vi "Navigation.vi"(0 "IA State Output in":T1, 7 "a1":dbl=10.0, 9 "a3":dbl=15.0, 11 "GoTo Navigation":bool, 12 "Debug":bool, 13 "output inc":dbl, 14 "output xy":dbl, 15 "output angle":dbl) -> (4 "IA State Output out":T1)   [LabVIEW 2018]
uses:
  Communication_class/Paths/MessageAI_State Folder/Intel/Command Enum.ctl
  Vision_class/Old vision/Controls/Functions Enum.ctl
  Utilities_class/Utilities.lvclass
  Vision_class/Old vision/Controls/AttackerStates.ctl
  Vision_class/Old vision/Controls/AI Robot.ctl
  Communication_class/Paths/MessageAI_State Folder/Core/AI Ball.ctl
  Communication_class/Paths/MessageAI_State Folder/Core/Field Size.ctl
  Communication_class/Paths/MessageAI_State Folder/Core/AI Judge.ctl
  Communication_class/Paths/MessageAI_State Folder/Util/Events/Events.ctl
  Communication_class/Paths/MessageAI_State Folder/Core/AI Input.ctl
  Vision_class/Old vision/Controls/PathDest.ctl
  Vision_class/Old vision/Controls/PathDests.ctl
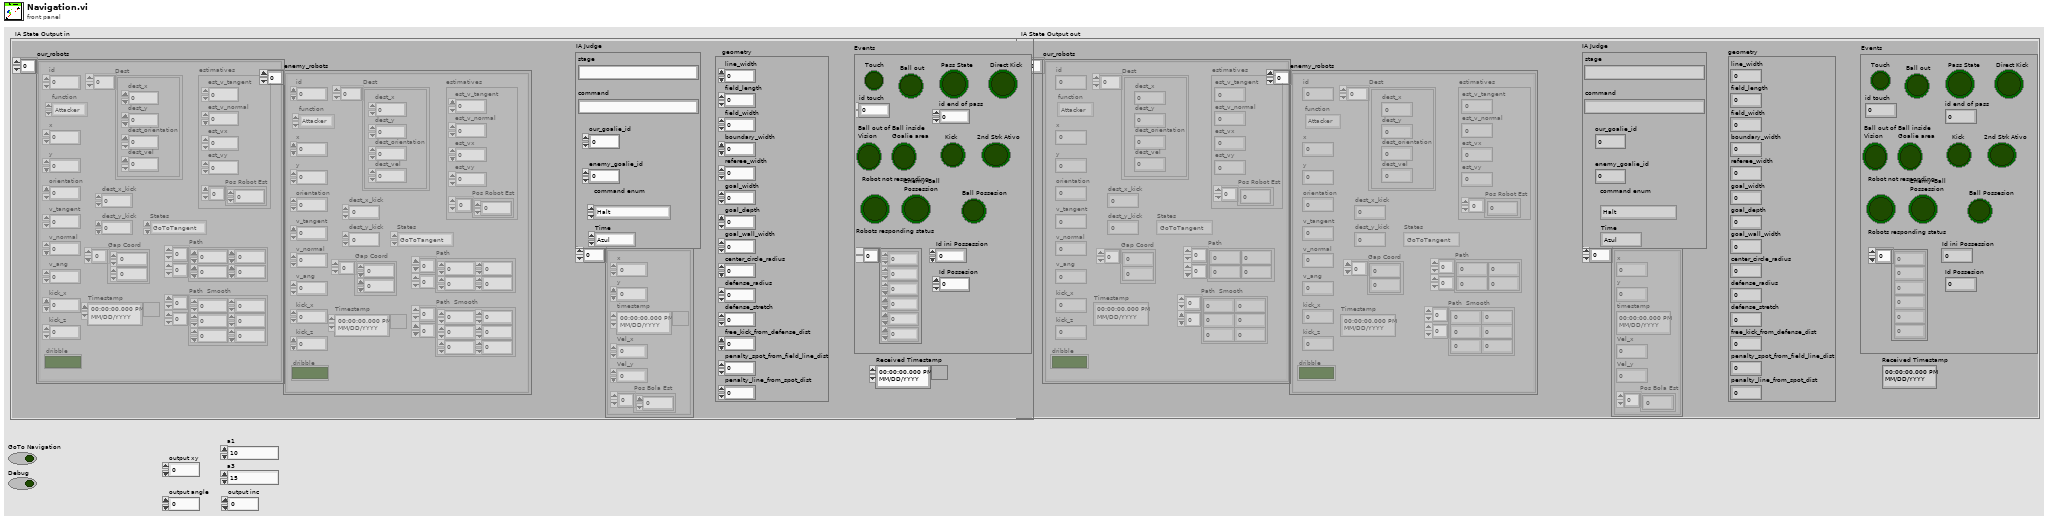
[diagram p1: front panel]
types:
  T1 = typedef "AI Input.ctl" = cluster{"our_robots":T2[], "enemy_robots":T2[], "balls":T7[], "geometry":T8, "IA Judge":T9, "Received Timestamp":timestamp, "Events":T11}
  T2 = typedef "AI Robot.ctl" = cluster{"id":u32, "function":T3, "x":dbl, "y":dbl, "orientation":dbl, "v_tangent":dbl, "v_normal":dbl, "v_ang":dbl, "kick_x":dbl, "kick_z":dbl, "dribble":bool, "Timestamp":timestamp, "estimatives":cluster{"est_v_tangent":dbl, "est_v_normal":dbl, "est_vx":dbl, "est_vy":dbl, "Pos Robot Est":dbl[]}, "dest_x_kick":dbl, "dest_y_kick":dbl, "Gap Coord":dbl[], "States":T4, "Path ":dbl[][], "Path  Smooth":dbl[][], "Dest":T5}
  T3 = typedef "Functions Enum.ctl" = enum16{"2nd Striker", "Attacker", "Goalie", "Defender", "Striker", "Goto 0", "Dummy", "Kicker", "ZigZag 0", "ZigZag 1", "ZigZag 2", "ZigZag 3", "ZigZag 4", "ZigZag 5", "ZigZag 6", "ZigZag 7", "ZigZag 8", ""}
  T4 = typedef "AttackerStates.ctl" = enum16{"Pass", "GoToTangent", "BallGetting", "GoToKick", ""}
  T5 = typedef "PathDests.ctl" = T6[]
  T6 = typedef "PathDest.ctl" = cluster{"dest_x":dbl, "dest_y":dbl, "dest_orientation":dbl, "dest_vel":dbl}
  T7 = typedef "AI Ball.ctl" = cluster{"x":dbl, "y":dbl, "timestamp":timestamp, "Vel_x":dbl, "Vel_y":dbl, "Pos Bola Est":dbl[]}
  T8 = typedef "Field Size.ctl" = cluster{"line_width":u32, "field_length":u32, "field_width":u32, "boundary_width":u32, "referee_width":u32, "goal_width":u32, "goal_depth":u32, "goal_wall_width":u32, "center_circle_radius":u32, "defense_radius":u32, "defense_stretch":u32, "free_kick_from_defense_dist":u32, "penalty_spot_from_field_line_dist":u32, "penalty_line_from_spot_dist":u32}
  T9 = typedef "AI Judge.ctl" = cluster{"stage":string, "command":string, "our_goalie_id":dbl, "enemy_goalie_id":dbl, "command enum":T10, "Time":enum16{"Azul", "Amarelo"}}
  T10 = typedef "Command Enum.ctl" = enum16{"Halt", "Stop", "Force Start", "PKA Normal Start", "Prepare Kickoff Ally", "PKE Normal Start", "Prepare Kickoff Enemy", "Prepare Penalty Ally", "PPA Normal Start", "Prepare Penalty Enemy", "PPE Normal Start", "Direct Free Enemy", "Direct Free Ally", "Indirect Free Enemy", "Indirect Free Ally", "Timeout Enemy", "Timeout Ally", "Goal Enemy", "Goal Ally", "Ball Placement Enemy", "Ball Placement Ally", "Normal Half Time", "Extra Time Break", "Extra Half Time", "None", "Post Game"}
  T11 = typedef "Events.ctl" = cluster{"Touch":bool, "Ball out":bool, "id touch":dbl, "Ball out of \nVision":bool, "Ball inside \nGoalie area":bool, "Robot not responding":bool, "Robots responding status":dbl[], "Enemy Ball \nPossession":bool, "Pass State":bool, "id end of pass":dbl, "Kick":bool, "Id ini Possession":dbl, "Ball Possesion":bool, "Id Possesion":dbl, "Direct Kick":bool, "2nd Strk Ativo":bool}
  T12 = cluster{"est_v_tangent":dbl, "est_v_normal":dbl, "est_vx":dbl, "est_vy":dbl, "Pos Robot Est":dbl[]}
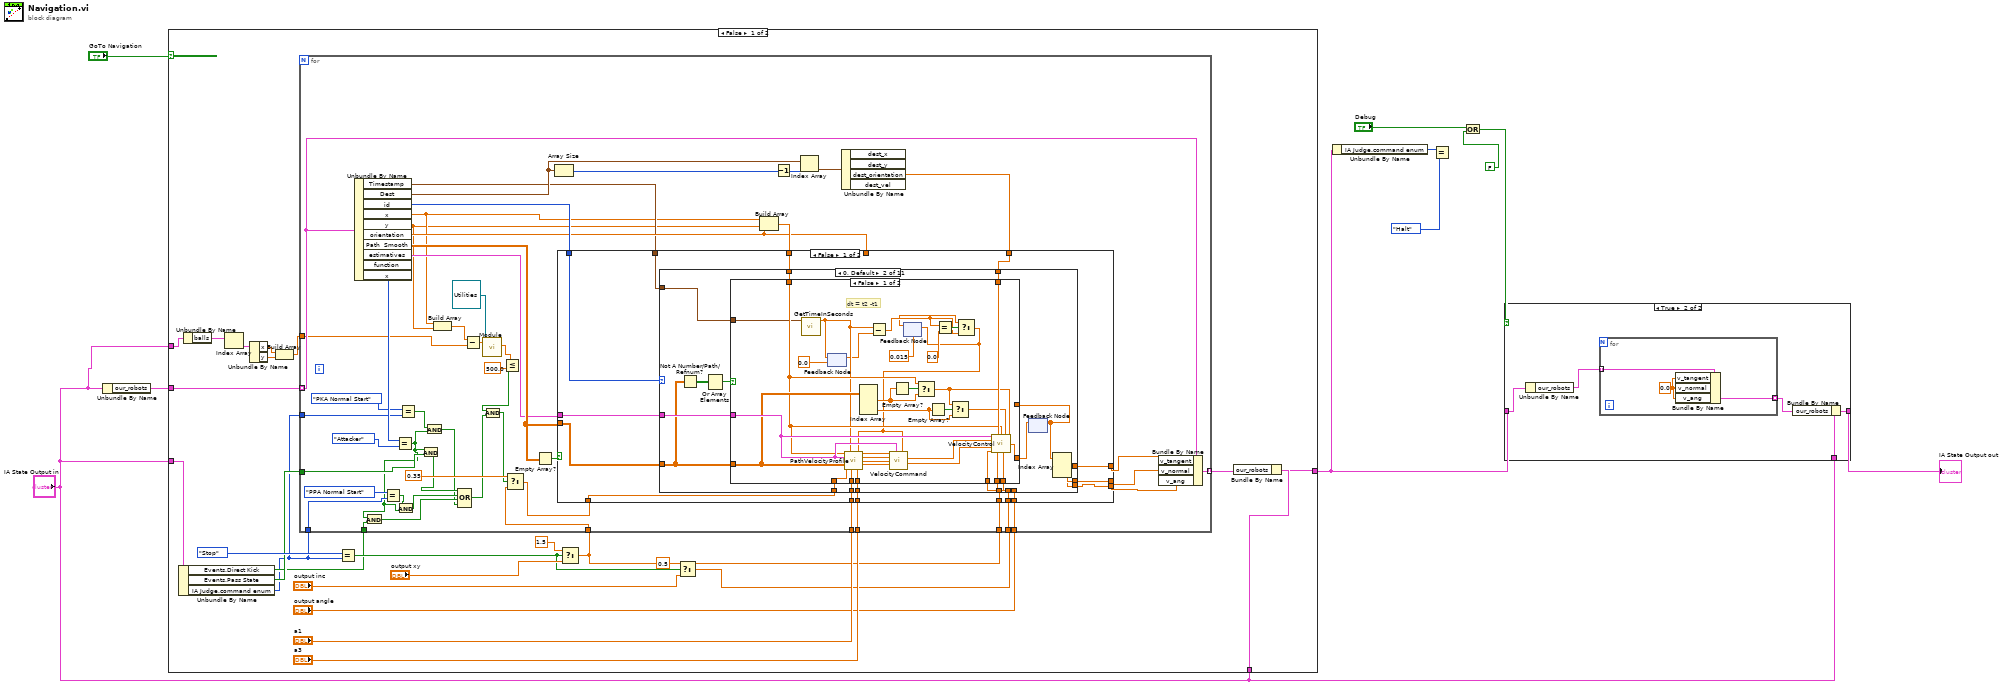
[diagram p0: block diagram]
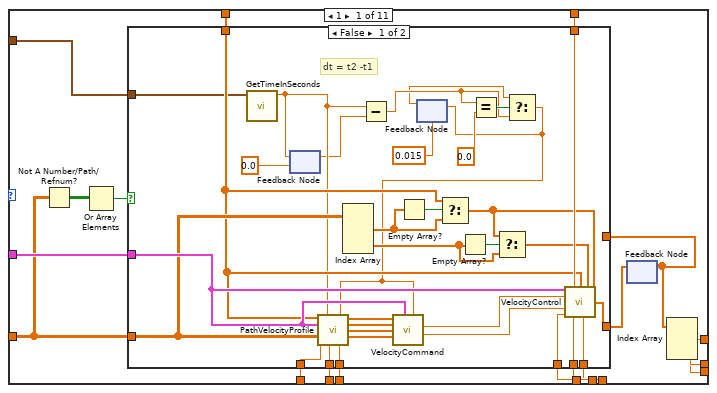
[diagram p2: hidden frame]
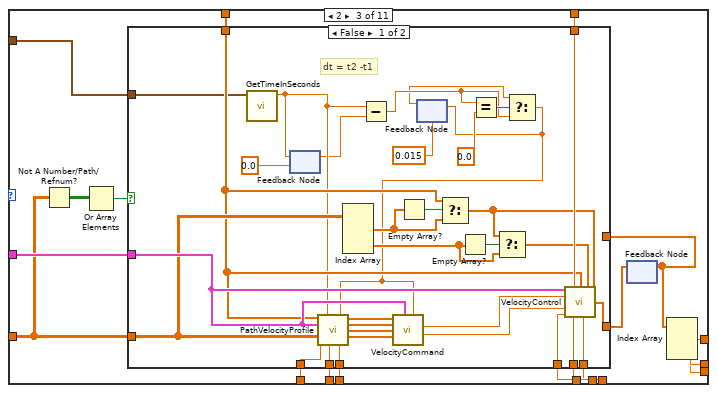
[diagram p5: hidden frame]
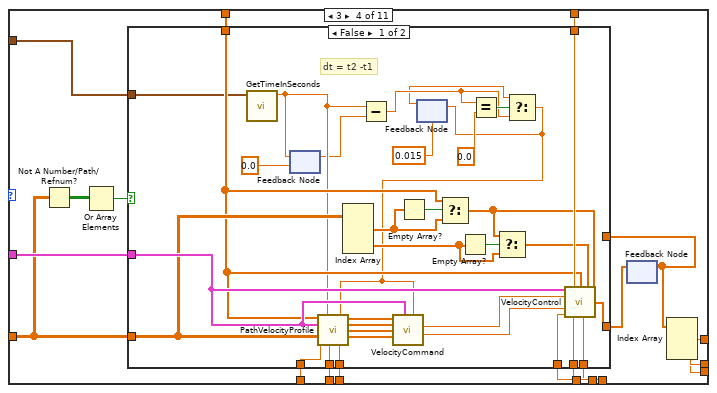
[diagram p7: hidden frame]
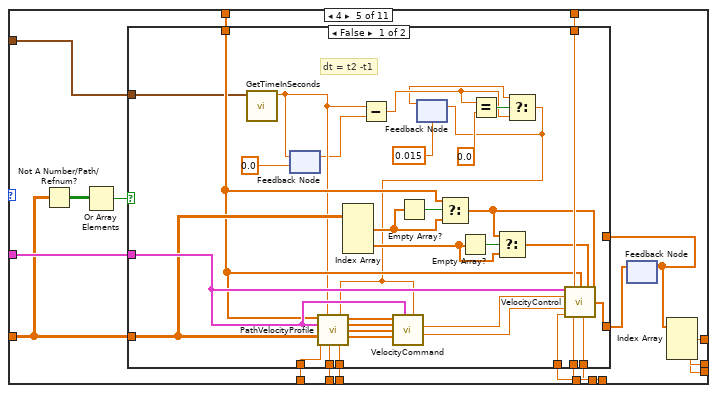
[diagram p9: hidden frame]
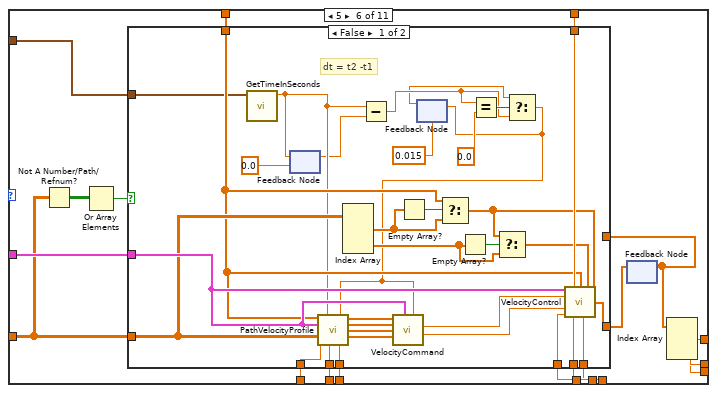
[diagram p11: hidden frame]
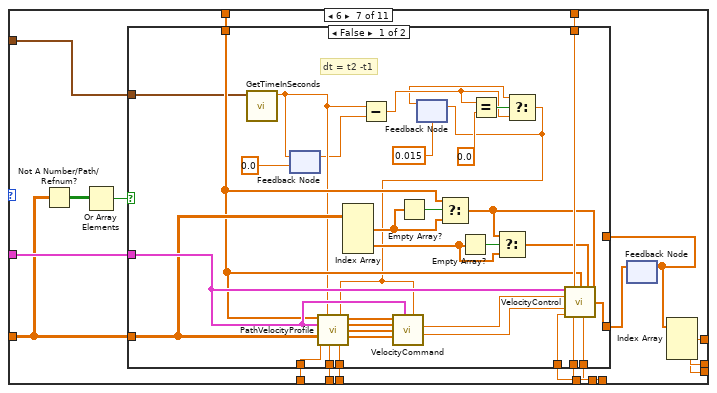
[diagram p13: hidden frame]
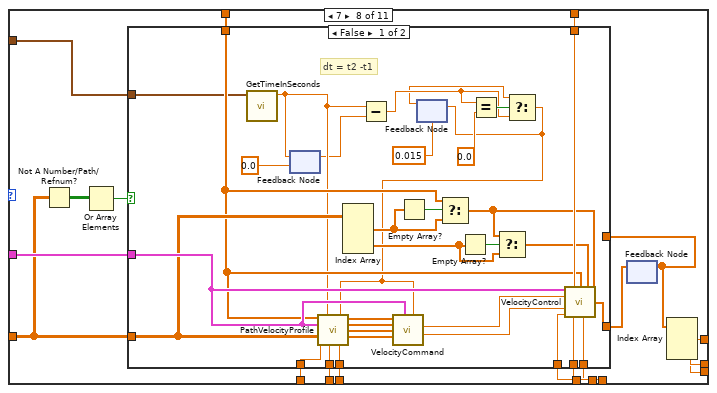
[diagram p15: hidden frame]
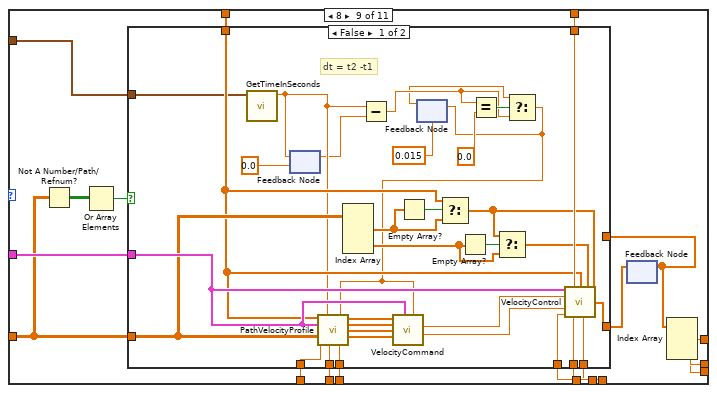
[diagram p17: hidden frame]
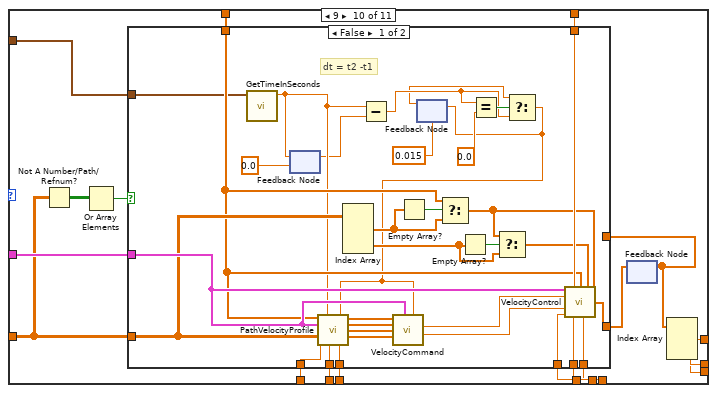
[diagram p19: hidden frame]
diagram:
  n1 = Unbundle By Name("IA State Output in") -> ("our_robots"=w10:T2[])
  n2 = case shown="False" "GoTo Navigation" {
    tunnel: w10 -> [w35 _]
    tunnel: [w32 w675] -> w7
    tunnel: "IA State Output in" -> [w28 w676]
    tunnel: "IA State Output in" -> [w33 _]
    tunnel: "IA State Output in" -> [w12 _]
    frame False {
      n3 = Unbundle By Name(w28) -> ("Events.Direct Kick"=w18:bool, "Events.Pass State"=w19:bool, "IA Judge.command enum"=w17:T10)
      n4 = Unbundle By Name(w12) -> ("balls"=w16:T7[])
      n5 = Index Array(array=w16) -> (element=w15:T7)  [unwired: 1 in]
      n6 = Unbundle By Name(w15) -> ("x"=w14:dbl, "y"=w13:dbl)
      n7 = Build Array(w14, w13) -> (w11:dbl[])
      n8 = Equal?(x=Command_Enum."Stop", y=w17) -> (x = y?=w23:bool)
      n9 = Select(t=1.5, s=w23, f="output xy") -> (s? t:f=w25:dbl)
      n10 = Select(t=0.5, s=w23, f="output inc") -> (s? t:f=w21:dbl)
      n11 = for {
        tunnel: w35 -> [w86] mode=indexing
        tunnel: [w85] -> w34 mode=indexing
        tunnel: w25 -> [w63]
        tunnel: "a1" -> [w74]
        tunnel: "a3" -> [w73]
        tunnel: w21 -> [w69]
        tunnel: "output angle" -> [w68]
        tunnel: w25 -> [w67]
        tunnel: w19 -> [w56]
        tunnel: w17 -> [w60]
        tunnel: w18 -> [w53]
        tunnel: w17 -> [w51]
        tunnel: w11 -> [w39]
        n12 = Unbundle By Name(w86) -> ("Timestamp"=w65:timestamp, "Dest"=w84:T5, "id"=w77:u32, "x"=w46:dbl, "y"=w45:dbl, "orientation"=w72:dbl, "Path  Smooth"=w78:dbl[][], "estimatives"=w75:T12, "function"=w52:T3)  [unwired: 1 out]
        n13 = Equal?(x=Command_Enum."PPA Normal Start", y=w60) -> (x = y?=w57:bool)
        n14 = Equal?(x=w52, y=Functions_Enum."Attacker") -> (x = y?=w48:bool)
        n15 = And(x=w48, y=w53) -> (x .and. y?=w54:bool)
        n16 = And(x=w57, y=w48) -> (x .and. y?=w55:bool)
        n17 = Equal?(x=Command_Enum."PKA Normal Start", y=w51) -> (x = y?=w49:bool)
        n18 = And(x=w48, y=w56) -> (x .and. y?=w58:bool)
        n19 = And(x=w49, y=w48) -> (x .and. y?=w47:bool)
        n20 = Build Array(w46, w45) -> (w40:dbl[])
        n21 = Compound Arithmetic op=OR(w58, w55, w54, w47) -> (w42:bool)
        n22 = Subtract(x=w40, y=w39) -> (x-y=w38:dbl[])
        n23 = call-dynamic "Module.vi"("2D vector"=w38, "Utilities in"=refnum<class "Utilities.lvclass"> refnum) -> ("Modulo"=w37:dbl)  [unwired: 7 in, 2 out]
        n24 = Less Or Equal?(x=w37, y=500.0) -> (x <= y?=w43:bool)
        n25 = And(x=w43, y=w42) -> (x .and. y?=w41:bool)
        n26 = Select(t=0.35, s=w41, f=w63) -> (s? t:f=w62:dbl)
        n27 = Empty Array?(array=w78) -> (empty?=w79:bool)
        n28 = Array Size(array=w84) -> (size(s)=w83:i32)
        n29 = Build Array(w46, w45, w72) -> (w76:dbl[])
        n30 = Decrement(x=w83) -> (x-1=w82:i32)
        n31 = Index Array(array=w84, index=w82) -> (element=w81:T6)
        n32 = Unbundle By Name(w81) -> ("dest_orientation"=w80:dbl)  [unwired: 3 out]
        n33 = case shown="False" w79 {
          tunnel: [w91 w674] -> w71
          tunnel: [w90 w674] -> w70
          tunnel: [w89 w674] -> w66
          tunnel: w77 -> [w87 _]
          tunnel: w78 -> [w93 _]
          tunnel: w80 -> [w94 _]
          tunnel: w76 -> [w92 _]
          tunnel: w75 -> [w95 _]
          tunnel: w62 -> [w101 _]
          tunnel: w74 -> [w100 _]
          tunnel: w73 -> [w99 _]
          tunnel: w72 -> [_ _]
          tunnel: w69 -> [w98 _]
          tunnel: w68 -> [w97 _]
          tunnel: w67 -> [w96 _]
          tunnel: w65 -> [w88 _]
          frame False {
            n34 = case shown="0, Default" w87 {
              tunnel: w101 -> [w119 w171 w223 w275 w327 w379 w431 w483 w535 w587 w639]
              tunnel: w100 -> [w118 w170 w222 w274 w326 w378 w430 w482 w534 w586 w638]
              tunnel: w99 -> [w117 w169 w221 w273 w325 w377 w429 w481 w533 w585 w637]
              tunnel: w98 -> [w116 w168 w220 w272 w324 w376 w428 w480 w532 w584 w636]
              tunnel: w97 -> [w115 w167 w219 w271 w323 w375 w427 w479 w531 w583 w635]
              tunnel: w96 -> [w114 w166 w218 w270 w322 w374 w426 w478 w530 w582 w634]
              tunnel: w95 -> [w113 w165 w217 w269 w321 w373 w425 w477 w529 w581 w633]
              tunnel: w94 -> [w112 w164 w216 w268 w320 w372 w424 w476 w528 w580 w632]
              tunnel: w93 -> [w104 w156 w208 w260 w312 w364 w416 w468 w520 w572 w624]
              tunnel: w92 -> [w111 w163 w215 w267 w319 w371 w423 w475 w527 w579 w631]
              tunnel: [w110 w162 w214 w266 w318 w370 w422 w474 w526 w578 w630] -> w91
              tunnel: [w109 w161 w213 w265 w317 w369 w421 w473 w525 w577 w629] -> w90
              tunnel: [w108 w160 w212 w264 w316 w368 w420 w472 w524 w576 w628] -> w89
              tunnel: w88 -> [w107 w159 w211 w263 w315 w367 w419 w471 w523 w575 w627]
              frame 1 {
                n35 = Not A Number/Path/Refnum?(number/path/refnum=w104) -> (NaN/Path/Refnum?=w103:bool[][])
                n36 = Or Array Elements(Boolean array=w103) -> (logical OR=w102:bool)
                n37 = feedback #1() -> (w105:dbl[])  [unwired: 1 in]
                n38 = case shown="False" w102 {
                  tunnel: w119 -> [w152 _]
                  tunnel: w118 -> [w151 _]
                  tunnel: w117 -> [w150 _]
                  tunnel: w116 -> [w149 _]
                  tunnel: w115 -> [w148 _]
                  tunnel: w114 -> [w147 _]
                  tunnel: w113 -> [w146 _]
                  tunnel: w112 -> [w145 _]
                  tunnel: w104 -> [w144 _]
                  tunnel: w111 -> [w143 _]
                  tunnel: [w142 w153] -> w106
                  tunnel: w107 -> [w129 _]
                  tunnel: w105 -> [_ w153]
                  frame False {
                    # "dt = t2 -t1"
                    n39 = call "GetTimeInSeconds.vi"("Timestamp"=w129) -> ("Numeric"=w123:dbl)  [unwired: 10 in]
                    n40 = feedback-in #2(w123) -> ()
                    n41 = feedback #2(0.0 ("Numeric")) -> (w122:dbl)
                    n42 = Index Array(array=w144) -> (element #1=w131:dbl[], element #2=w134:dbl[])  [unwired: 4 in]
                    n43 = Subtract(x=w123, y=w122) -> (x-y=w125:dbl)
                    n44 = Empty Array?(array=w131) -> (empty?=w132:bool)
                    n45 = feedback #3(0.015 ("Numeric")) -> (w124:dbl)
                    n46 = Select(t=w143, s=w132, f=w131) -> (s? t:f=w130:dbl[])
                    n47 = Empty Array?(array=w134) -> (empty?=w135:bool)
                    n48 = Equal?(x=w125, y=0.0) -> (x = y?=w128:bool)
                    n49 = Select(t=w130, s=w135, f=w134) -> (s? t:f=w133:dbl[])
                    n50 = Select(t=w124, s=w128, f=w125) -> (s? t:f=w120:dbl)
                    n51 = call "PathVelocityProfile.vi"("Pose"=w143, "time"=w123, "intervalo"=w120, "estimatives"=w146, "Path  Smooth"=w144, "V_max"=w152, "Accel"=w151, "DesAccel"=w150) -> ("Time X"=w141:dbl[], "Velocities X"=w140:dbl[], "Time Y"=w139:dbl[], "Velocities Y"=w138:dbl[])  [unwired: 4 in]
                    n52 = call "VelocityCommand.vi"("intervalo"=w120, "estimatives"=w146, "Velocities Y"=w138, "Time Y"=w139, "Velocities X"=w140, "Time X"=w141) -> ("Vy"=w137:dbl, "Vx"=w136:dbl)  [unwired: 4 in]
                    n53 = feedback-in #3(w120) -> ()
                    n54 = call "VelocityControl.vi"("estimatives"=w146, "Dest_orientation"=w145, "Position"=w143, "Waypoint 1"=w133, "Waypoint 0"=w130, "Vx"=w136, "Vy"=w137, "output xy"=w147, "output inc"=w149, "output angle"=w148) -> ("Output Velocity"=w142:dbl[])  [unwired: 5 in]
                  }
                  frame True {
                  }
                }
                n55 = feedback-in #1(w106) -> ()
                n56 = Index Array(array=w105) -> (element #1=w110:dbl, element #2=w109:dbl, element #3=w108:dbl)  [unwired: 3 in]
              }
              frame 0, Default {
                n57 = Not A Number/Path/Refnum?(number/path/refnum=w156) -> (NaN/Path/Refnum?=w155:bool[][])
                n58 = Or Array Elements(Boolean array=w155) -> (logical OR=w154:bool)
                n59 = feedback #4() -> (w157:dbl[])  [unwired: 1 in]
                n60 = case shown="False" w154 {
                  tunnel: w171 -> [w204 _]
                  tunnel: w170 -> [w203 _]
                  tunnel: w169 -> [w202 _]
                  tunnel: w168 -> [w201 _]
                  tunnel: w167 -> [w200 _]
                  tunnel: w166 -> [w199 _]
                  tunnel: w165 -> [w198 _]
                  tunnel: w164 -> [w197 _]
                  tunnel: w156 -> [w196 _]
                  tunnel: w163 -> [w195 _]
                  tunnel: [w194 w205] -> w158
                  tunnel: w159 -> [w181 _]
                  tunnel: w157 -> [_ w205]
                  frame False {
                    # "dt = t2 -t1"
                    n61 = call "GetTimeInSeconds.vi"("Timestamp"=w181) -> ("Numeric"=w175:dbl)  [unwired: 10 in]
                    n62 = feedback-in #5(w175) -> ()
                    n63 = feedback #5(0.0 ("Numeric")) -> (w174:dbl)
                    n64 = Index Array(array=w196) -> (element #1=w183:dbl[], element #2=w186:dbl[])  [unwired: 4 in]
                    n65 = Subtract(x=w175, y=w174) -> (x-y=w177:dbl)
                    n66 = Empty Array?(array=w183) -> (empty?=w184:bool)
                    n67 = feedback #6(0.015 ("Numeric")) -> (w176:dbl)
                    n68 = Select(t=w195, s=w184, f=w183) -> (s? t:f=w182:dbl[])
                    n69 = Empty Array?(array=w186) -> (empty?=w187:bool)
                    n70 = Equal?(x=w177, y=0.0) -> (x = y?=w180:bool)
                    n71 = Select(t=w182, s=w187, f=w186) -> (s? t:f=w185:dbl[])
                    n72 = Select(t=w176, s=w180, f=w177) -> (s? t:f=w172:dbl)
                    n73 = call "PathVelocityProfile.vi"("Pose"=w195, "time"=w175, "intervalo"=w172, "estimatives"=w198, "Path  Smooth"=w196, "V_max"=w204, "Accel"=w203, "DesAccel"=w202) -> ("Time X"=w193:dbl[], "Velocities X"=w192:dbl[], "Time Y"=w191:dbl[], "Velocities Y"=w190:dbl[])  [unwired: 4 in]
                    n74 = call "VelocityCommand.vi"("intervalo"=w172, "estimatives"=w198, "Velocities Y"=w190, "Time Y"=w191, "Velocities X"=w192, "Time X"=w193) -> ("Vy"=w189:dbl, "Vx"=w188:dbl)  [unwired: 4 in]
                    n75 = feedback-in #6(w172) -> ()
                    n76 = call "VelocityControl.vi"("estimatives"=w198, "Dest_orientation"=w197, "Position"=w195, "Waypoint 1"=w185, "Waypoint 0"=w182, "Vx"=w188, "Vy"=w189, "output xy"=w199, "output inc"=w201, "output angle"=w200) -> ("Output Velocity"=w194:dbl[])  [unwired: 5 in]
                  }
                  frame True {
                  }
                }
                n77 = feedback-in #4(w158) -> ()
                n78 = Index Array(array=w157) -> (element #1=w162:dbl, element #2=w161:dbl, element #3=w160:dbl)  [unwired: 3 in]
              }
              frame 2 {
                n79 = Not A Number/Path/Refnum?(number/path/refnum=w208) -> (NaN/Path/Refnum?=w207:bool[][])
                n80 = Or Array Elements(Boolean array=w207) -> (logical OR=w206:bool)
                n81 = feedback #7() -> (w209:dbl[])  [unwired: 1 in]
                n82 = case shown="False" w206 {
                  tunnel: w223 -> [w256 _]
                  tunnel: w222 -> [w255 _]
                  tunnel: w221 -> [w254 _]
                  tunnel: w220 -> [w253 _]
                  tunnel: w219 -> [w252 _]
                  tunnel: w218 -> [w251 _]
                  tunnel: w217 -> [w250 _]
                  tunnel: w216 -> [w249 _]
                  tunnel: w208 -> [w248 _]
                  tunnel: w215 -> [w247 _]
                  tunnel: [w246 w257] -> w210
                  tunnel: w211 -> [w233 _]
                  tunnel: w209 -> [_ w257]
                  frame False {
                    # "dt = t2 -t1"
                    n83 = call "GetTimeInSeconds.vi"("Timestamp"=w233) -> ("Numeric"=w227:dbl)  [unwired: 10 in]
                    n84 = feedback-in #8(w227) -> ()
                    n85 = feedback #8(0.0 ("Numeric")) -> (w226:dbl)
                    n86 = Index Array(array=w248) -> (element #1=w235:dbl[], element #2=w238:dbl[])  [unwired: 4 in]
                    n87 = Subtract(x=w227, y=w226) -> (x-y=w229:dbl)
                    n88 = Empty Array?(array=w235) -> (empty?=w236:bool)
                    n89 = feedback #9(0.015 ("Numeric")) -> (w228:dbl)
                    n90 = Select(t=w247, s=w236, f=w235) -> (s? t:f=w234:dbl[])
                    n91 = Empty Array?(array=w238) -> (empty?=w239:bool)
                    n92 = Equal?(x=w229, y=0.0) -> (x = y?=w232:bool)
                    n93 = Select(t=w234, s=w239, f=w238) -> (s? t:f=w237:dbl[])
                    n94 = Select(t=w228, s=w232, f=w229) -> (s? t:f=w224:dbl)
                    n95 = call "PathVelocityProfile.vi"("Pose"=w247, "time"=w227, "intervalo"=w224, "estimatives"=w250, "Path  Smooth"=w248, "V_max"=w256, "Accel"=w255, "DesAccel"=w254) -> ("Time X"=w245:dbl[], "Velocities X"=w244:dbl[], "Time Y"=w243:dbl[], "Velocities Y"=w242:dbl[])  [unwired: 4 in]
                    n96 = call "VelocityCommand.vi"("intervalo"=w224, "estimatives"=w250, "Velocities Y"=w242, "Time Y"=w243, "Velocities X"=w244, "Time X"=w245) -> ("Vy"=w241:dbl, "Vx"=w240:dbl)  [unwired: 4 in]
                    n97 = feedback-in #9(w224) -> ()
                    n98 = call "VelocityControl.vi"("estimatives"=w250, "Dest_orientation"=w249, "Position"=w247, "Waypoint 1"=w237, "Waypoint 0"=w234, "Vx"=w240, "Vy"=w241, "output xy"=w251, "output inc"=w253, "output angle"=w252) -> ("Output Velocity"=w246:dbl[])  [unwired: 5 in]
                  }
                  frame True {
                  }
                }
                n99 = feedback-in #7(w210) -> ()
                n100 = Index Array(array=w209) -> (element #1=w214:dbl, element #2=w213:dbl, element #3=w212:dbl)  [unwired: 3 in]
              }
              frame 3 {
                n101 = Not A Number/Path/Refnum?(number/path/refnum=w260) -> (NaN/Path/Refnum?=w259:bool[][])
                n102 = Or Array Elements(Boolean array=w259) -> (logical OR=w258:bool)
                n103 = feedback #10() -> (w261:dbl[])  [unwired: 1 in]
                n104 = case shown="False" w258 {
                  tunnel: w275 -> [w308 _]
                  tunnel: w274 -> [w307 _]
                  tunnel: w273 -> [w306 _]
                  tunnel: w272 -> [w305 _]
                  tunnel: w271 -> [w304 _]
                  tunnel: w270 -> [w303 _]
                  tunnel: w269 -> [w302 _]
                  tunnel: w268 -> [w301 _]
                  tunnel: w260 -> [w300 _]
                  tunnel: w267 -> [w299 _]
                  tunnel: [w298 w309] -> w262
                  tunnel: w263 -> [w285 _]
                  tunnel: w261 -> [_ w309]
                  frame False {
                    # "dt = t2 -t1"
                    n105 = call "GetTimeInSeconds.vi"("Timestamp"=w285) -> ("Numeric"=w279:dbl)  [unwired: 10 in]
                    n106 = feedback-in #11(w279) -> ()
                    n107 = feedback #11(0.0 ("Numeric")) -> (w278:dbl)
                    n108 = Index Array(array=w300) -> (element #1=w287:dbl[], element #2=w290:dbl[])  [unwired: 4 in]
                    n109 = Subtract(x=w279, y=w278) -> (x-y=w281:dbl)
                    n110 = Empty Array?(array=w287) -> (empty?=w288:bool)
                    n111 = feedback #12(0.015 ("Numeric")) -> (w280:dbl)
                    n112 = Select(t=w299, s=w288, f=w287) -> (s? t:f=w286:dbl[])
                    n113 = Empty Array?(array=w290) -> (empty?=w291:bool)
                    n114 = Equal?(x=w281, y=0.0) -> (x = y?=w284:bool)
                    n115 = Select(t=w286, s=w291, f=w290) -> (s? t:f=w289:dbl[])
                    n116 = Select(t=w280, s=w284, f=w281) -> (s? t:f=w276:dbl)
                    n117 = call "PathVelocityProfile.vi"("Pose"=w299, "time"=w279, "intervalo"=w276, "estimatives"=w302, "Path  Smooth"=w300, "V_max"=w308, "Accel"=w307, "DesAccel"=w306) -> ("Time X"=w297:dbl[], "Velocities X"=w296:dbl[], "Time Y"=w295:dbl[], "Velocities Y"=w294:dbl[])  [unwired: 4 in]
                    n118 = call "VelocityCommand.vi"("intervalo"=w276, "estimatives"=w302, "Velocities Y"=w294, "Time Y"=w295, "Velocities X"=w296, "Time X"=w297) -> ("Vy"=w293:dbl, "Vx"=w292:dbl)  [unwired: 4 in]
                    n119 = feedback-in #12(w276) -> ()
                    n120 = call "VelocityControl.vi"("estimatives"=w302, "Dest_orientation"=w301, "Position"=w299, "Waypoint 1"=w289, "Waypoint 0"=w286, "Vx"=w292, "Vy"=w293, "output xy"=w303, "output inc"=w305, "output angle"=w304) -> ("Output Velocity"=w298:dbl[])  [unwired: 5 in]
                  }
                  frame True {
                  }
                }
                n121 = feedback-in #10(w262) -> ()
                n122 = Index Array(array=w261) -> (element #1=w266:dbl, element #2=w265:dbl, element #3=w264:dbl)  [unwired: 3 in]
              }
              frame 4 {
                n123 = Not A Number/Path/Refnum?(number/path/refnum=w312) -> (NaN/Path/Refnum?=w311:bool[][])
                n124 = Or Array Elements(Boolean array=w311) -> (logical OR=w310:bool)
                n125 = feedback #13() -> (w313:dbl[])  [unwired: 1 in]
                n126 = case shown="False" w310 {
                  tunnel: w327 -> [w360 _]
                  tunnel: w326 -> [w359 _]
                  tunnel: w325 -> [w358 _]
                  tunnel: w324 -> [w357 _]
                  tunnel: w323 -> [w356 _]
                  tunnel: w322 -> [w355 _]
                  tunnel: w321 -> [w354 _]
                  tunnel: w320 -> [w353 _]
                  tunnel: w312 -> [w352 _]
                  tunnel: w319 -> [w351 _]
                  tunnel: [w350 w361] -> w314
                  tunnel: w315 -> [w337 _]
                  tunnel: w313 -> [_ w361]
                  frame False {
                    # "dt = t2 -t1"
                    n127 = call "GetTimeInSeconds.vi"("Timestamp"=w337) -> ("Numeric"=w331:dbl)  [unwired: 10 in]
                    n128 = feedback-in #14(w331) -> ()
                    n129 = feedback #14(0.0 ("Numeric")) -> (w330:dbl)
                    n130 = Index Array(array=w352) -> (element #1=w339:dbl[], element #2=w342:dbl[])  [unwired: 4 in]
                    n131 = Subtract(x=w331, y=w330) -> (x-y=w333:dbl)
                    n132 = Empty Array?(array=w339) -> (empty?=w340:bool)
                    n133 = feedback #15(0.015 ("Numeric")) -> (w332:dbl)
                    n134 = Select(t=w351, s=w340, f=w339) -> (s? t:f=w338:dbl[])
                    n135 = Empty Array?(array=w342) -> (empty?=w343:bool)
                    n136 = Equal?(x=w333, y=0.0) -> (x = y?=w336:bool)
                    n137 = Select(t=w338, s=w343, f=w342) -> (s? t:f=w341:dbl[])
                    n138 = Select(t=w332, s=w336, f=w333) -> (s? t:f=w328:dbl)
                    n139 = call "PathVelocityProfile.vi"("Pose"=w351, "time"=w331, "intervalo"=w328, "estimatives"=w354, "Path  Smooth"=w352, "V_max"=w360, "Accel"=w359, "DesAccel"=w358) -> ("Time X"=w349:dbl[], "Velocities X"=w348:dbl[], "Time Y"=w347:dbl[], "Velocities Y"=w346:dbl[])  [unwired: 4 in]
                    n140 = call "VelocityCommand.vi"("intervalo"=w328, "estimatives"=w354, "Velocities Y"=w346, "Time Y"=w347, "Velocities X"=w348, "Time X"=w349) -> ("Vy"=w345:dbl, "Vx"=w344:dbl)  [unwired: 4 in]
                    n141 = feedback-in #15(w328) -> ()
                    n142 = call "VelocityControl.vi"("estimatives"=w354, "Dest_orientation"=w353, "Position"=w351, "Waypoint 1"=w341, "Waypoint 0"=w338, "Vx"=w344, "Vy"=w345, "output xy"=w355, "output inc"=w357, "output angle"=w356) -> ("Output Velocity"=w350:dbl[])  [unwired: 5 in]
                  }
                  frame True {
                  }
                }
                n143 = feedback-in #13(w314) -> ()
                n144 = Index Array(array=w313) -> (element #1=w318:dbl, element #2=w317:dbl, element #3=w316:dbl)  [unwired: 3 in]
              }
              frame 5 {
                n145 = Not A Number/Path/Refnum?(number/path/refnum=w364) -> (NaN/Path/Refnum?=w363:bool[][])
                n146 = Or Array Elements(Boolean array=w363) -> (logical OR=w362:bool)
                n147 = feedback #16() -> (w365:dbl[])  [unwired: 1 in]
                n148 = case shown="False" w362 {
                  tunnel: w379 -> [w412 _]
                  tunnel: w378 -> [w411 _]
                  tunnel: w377 -> [w410 _]
                  tunnel: w376 -> [w409 _]
                  tunnel: w375 -> [w408 _]
                  tunnel: w374 -> [w407 _]
                  tunnel: w373 -> [w406 _]
                  tunnel: w372 -> [w405 _]
                  tunnel: w364 -> [w404 _]
                  tunnel: w371 -> [w403 _]
                  tunnel: [w402 w413] -> w366
                  tunnel: w367 -> [w389 _]
                  tunnel: w365 -> [_ w413]
                  frame False {
                    # "dt = t2 -t1"
                    n149 = call "GetTimeInSeconds.vi"("Timestamp"=w389) -> ("Numeric"=w383:dbl)  [unwired: 10 in]
                    n150 = feedback-in #17(w383) -> ()
                    n151 = feedback #17(0.0 ("Numeric")) -> (w382:dbl)
                    n152 = Index Array(array=w404) -> (element #1=w391:dbl[], element #2=w394:dbl[])  [unwired: 4 in]
                    n153 = Subtract(x=w383, y=w382) -> (x-y=w385:dbl)
                    n154 = Empty Array?(array=w391) -> (empty?=w392:bool)
                    n155 = feedback #18(0.015 ("Numeric")) -> (w384:dbl)
                    n156 = Select(t=w403, s=w392, f=w391) -> (s? t:f=w390:dbl[])
                    n157 = Empty Array?(array=w394) -> (empty?=w395:bool)
                    n158 = Equal?(x=w385, y=0.0) -> (x = y?=w388:bool)
                    n159 = Select(t=w390, s=w395, f=w394) -> (s? t:f=w393:dbl[])
                    n160 = Select(t=w384, s=w388, f=w385) -> (s? t:f=w380:dbl)
                    n161 = call "PathVelocityProfile.vi"("Pose"=w403, "time"=w383, "intervalo"=w380, "estimatives"=w406, "Path  Smooth"=w404, "V_max"=w412, "Accel"=w411, "DesAccel"=w410) -> ("Time X"=w401:dbl[], "Velocities X"=w400:dbl[], "Time Y"=w399:dbl[], "Velocities Y"=w398:dbl[])  [unwired: 4 in]
                    n162 = call "VelocityCommand.vi"("intervalo"=w380, "estimatives"=w406, "Velocities Y"=w398, "Time Y"=w399, "Velocities X"=w400, "Time X"=w401) -> ("Vy"=w397:dbl, "Vx"=w396:dbl)  [unwired: 4 in]
                    n163 = feedback-in #18(w380) -> ()
                    n164 = call "VelocityControl.vi"("estimatives"=w406, "Dest_orientation"=w405, "Position"=w403, "Waypoint 1"=w393, "Waypoint 0"=w390, "Vx"=w396, "Vy"=w397, "output xy"=w407, "output inc"=w409, "output angle"=w408) -> ("Output Velocity"=w402:dbl[])  [unwired: 5 in]
                  }
                  frame True {
                  }
                }
                n165 = feedback-in #16(w366) -> ()
                n166 = Index Array(array=w365) -> (element #1=w370:dbl, element #2=w369:dbl, element #3=w368:dbl)  [unwired: 3 in]
              }
              frame 6 {
                n167 = Not A Number/Path/Refnum?(number/path/refnum=w416) -> (NaN/Path/Refnum?=w415:bool[][])
                n168 = Or Array Elements(Boolean array=w415) -> (logical OR=w414:bool)
                n169 = feedback #19() -> (w417:dbl[])  [unwired: 1 in]
                n170 = case shown="False" w414 {
                  tunnel: w431 -> [w464 _]
                  tunnel: w430 -> [w463 _]
                  tunnel: w429 -> [w462 _]
                  tunnel: w428 -> [w461 _]
                  tunnel: w427 -> [w460 _]
                  tunnel: w426 -> [w459 _]
                  tunnel: w425 -> [w458 _]
                  tunnel: w424 -> [w457 _]
                  tunnel: w416 -> [w456 _]
                  tunnel: w423 -> [w455 _]
                  tunnel: [w454 w465] -> w418
                  tunnel: w419 -> [w441 _]
                  tunnel: w417 -> [_ w465]
                  frame False {
                    # "dt = t2 -t1"
                    n171 = call "GetTimeInSeconds.vi"("Timestamp"=w441) -> ("Numeric"=w435:dbl)  [unwired: 10 in]
                    n172 = feedback-in #20(w435) -> ()
                    n173 = feedback #20(0.0 ("Numeric")) -> (w434:dbl)
                    n174 = Index Array(array=w456) -> (element #1=w443:dbl[], element #2=w446:dbl[])  [unwired: 4 in]
                    n175 = Subtract(x=w435, y=w434) -> (x-y=w437:dbl)
                    n176 = Empty Array?(array=w443) -> (empty?=w444:bool)
                    n177 = feedback #21(0.015 ("Numeric")) -> (w436:dbl)
                    n178 = Select(t=w455, s=w444, f=w443) -> (s? t:f=w442:dbl[])
                    n179 = Empty Array?(array=w446) -> (empty?=w447:bool)
                    n180 = Equal?(x=w437, y=0.0) -> (x = y?=w440:bool)
                    n181 = Select(t=w442, s=w447, f=w446) -> (s? t:f=w445:dbl[])
                    n182 = Select(t=w436, s=w440, f=w437) -> (s? t:f=w432:dbl)
                    n183 = call "PathVelocityProfile.vi"("Pose"=w455, "time"=w435, "intervalo"=w432, "estimatives"=w458, "Path  Smooth"=w456, "V_max"=w464, "Accel"=w463, "DesAccel"=w462) -> ("Time X"=w453:dbl[], "Velocities X"=w452:dbl[], "Time Y"=w451:dbl[], "Velocities Y"=w450:dbl[])  [unwired: 4 in]
                    n184 = call "VelocityCommand.vi"("intervalo"=w432, "estimatives"=w458, "Velocities Y"=w450, "Time Y"=w451, "Velocities X"=w452, "Time X"=w453) -> ("Vy"=w449:dbl, "Vx"=w448:dbl)  [unwired: 4 in]
                    n185 = feedback-in #21(w432) -> ()
                    n186 = call "VelocityControl.vi"("estimatives"=w458, "Dest_orientation"=w457, "Position"=w455, "Waypoint 1"=w445, "Waypoint 0"=w442, "Vx"=w448, "Vy"=w449, "output xy"=w459, "output inc"=w461, "output angle"=w460) -> ("Output Velocity"=w454:dbl[])  [unwired: 5 in]
                  }
                  frame True {
                  }
                }
                n187 = feedback-in #19(w418) -> ()
                n188 = Index Array(array=w417) -> (element #1=w422:dbl, element #2=w421:dbl, element #3=w420:dbl)  [unwired: 3 in]
              }
              frame 7 {
                n189 = Not A Number/Path/Refnum?(number/path/refnum=w468) -> (NaN/Path/Refnum?=w467:bool[][])
                n190 = Or Array Elements(Boolean array=w467) -> (logical OR=w466:bool)
                n191 = feedback #22() -> (w469:dbl[])  [unwired: 1 in]
                n192 = case shown="False" w466 {
                  tunnel: w483 -> [w516 _]
                  tunnel: w482 -> [w515 _]
                  tunnel: w481 -> [w514 _]
                  tunnel: w480 -> [w513 _]
                  tunnel: w479 -> [w512 _]
                  tunnel: w478 -> [w511 _]
                  tunnel: w477 -> [w510 _]
                  tunnel: w476 -> [w509 _]
                  tunnel: w468 -> [w508 _]
                  tunnel: w475 -> [w507 _]
                  tunnel: [w506 w517] -> w470
                  tunnel: w471 -> [w493 _]
                  tunnel: w469 -> [_ w517]
                  frame False {
                    # "dt = t2 -t1"
                    n193 = call "GetTimeInSeconds.vi"("Timestamp"=w493) -> ("Numeric"=w487:dbl)  [unwired: 10 in]
                    n194 = feedback-in #23(w487) -> ()
                    n195 = feedback #23(0.0 ("Numeric")) -> (w486:dbl)
                    n196 = Index Array(array=w508) -> (element #1=w495:dbl[], element #2=w498:dbl[])  [unwired: 4 in]
                    n197 = Subtract(x=w487, y=w486) -> (x-y=w489:dbl)
                    n198 = Empty Array?(array=w495) -> (empty?=w496:bool)
                    n199 = feedback #24(0.015 ("Numeric")) -> (w488:dbl)
                    n200 = Select(t=w507, s=w496, f=w495) -> (s? t:f=w494:dbl[])
                    n201 = Empty Array?(array=w498) -> (empty?=w499:bool)
                    n202 = Equal?(x=w489, y=0.0) -> (x = y?=w492:bool)
                    n203 = Select(t=w494, s=w499, f=w498) -> (s? t:f=w497:dbl[])
                    n204 = Select(t=w488, s=w492, f=w489) -> (s? t:f=w484:dbl)
                    n205 = call "PathVelocityProfile.vi"("Pose"=w507, "time"=w487, "intervalo"=w484, "estimatives"=w510, "Path  Smooth"=w508, "V_max"=w516, "Accel"=w515, "DesAccel"=w514) -> ("Time X"=w505:dbl[], "Velocities X"=w504:dbl[], "Time Y"=w503:dbl[], "Velocities Y"=w502:dbl[])  [unwired: 4 in]
                    n206 = call "VelocityCommand.vi"("intervalo"=w484, "estimatives"=w510, "Velocities Y"=w502, "Time Y"=w503, "Velocities X"=w504, "Time X"=w505) -> ("Vy"=w501:dbl, "Vx"=w500:dbl)  [unwired: 4 in]
                    n207 = feedback-in #24(w484) -> ()
                    n208 = call "VelocityControl.vi"("estimatives"=w510, "Dest_orientation"=w509, "Position"=w507, "Waypoint 1"=w497, "Waypoint 0"=w494, "Vx"=w500, "Vy"=w501, "output xy"=w511, "output inc"=w513, "output angle"=w512) -> ("Output Velocity"=w506:dbl[])  [unwired: 5 in]
                  }
                  frame True {
                  }
                }
                n209 = feedback-in #22(w470) -> ()
                n210 = Index Array(array=w469) -> (element #1=w474:dbl, element #2=w473:dbl, element #3=w472:dbl)  [unwired: 3 in]
              }
              frame 8 {
                n211 = Not A Number/Path/Refnum?(number/path/refnum=w520) -> (NaN/Path/Refnum?=w519:bool[][])
                n212 = Or Array Elements(Boolean array=w519) -> (logical OR=w518:bool)
                n213 = feedback #25() -> (w521:dbl[])  [unwired: 1 in]
                n214 = case shown="False" w518 {
                  tunnel: w535 -> [w568 _]
                  tunnel: w534 -> [w567 _]
                  tunnel: w533 -> [w566 _]
                  tunnel: w532 -> [w565 _]
                  tunnel: w531 -> [w564 _]
                  tunnel: w530 -> [w563 _]
                  tunnel: w529 -> [w562 _]
                  tunnel: w528 -> [w561 _]
                  tunnel: w520 -> [w560 _]
                  tunnel: w527 -> [w559 _]
                  tunnel: [w558 w569] -> w522
                  tunnel: w523 -> [w545 _]
                  tunnel: w521 -> [_ w569]
                  frame False {
                    # "dt = t2 -t1"
                    n215 = call "GetTimeInSeconds.vi"("Timestamp"=w545) -> ("Numeric"=w539:dbl)  [unwired: 10 in]
                    n216 = feedback-in #26(w539) -> ()
                    n217 = feedback #26(0.0 ("Numeric")) -> (w538:dbl)
                    n218 = Index Array(array=w560) -> (element #1=w547:dbl[], element #2=w550:dbl[])  [unwired: 4 in]
                    n219 = Subtract(x=w539, y=w538) -> (x-y=w541:dbl)
                    n220 = Empty Array?(array=w547) -> (empty?=w548:bool)
                    n221 = feedback #27(0.015 ("Numeric")) -> (w540:dbl)
                    n222 = Select(t=w559, s=w548, f=w547) -> (s? t:f=w546:dbl[])
                    n223 = Empty Array?(array=w550) -> (empty?=w551:bool)
                    n224 = Equal?(x=w541, y=0.0) -> (x = y?=w544:bool)
                    n225 = Select(t=w546, s=w551, f=w550) -> (s? t:f=w549:dbl[])
                    n226 = Select(t=w540, s=w544, f=w541) -> (s? t:f=w536:dbl)
                    n227 = call "PathVelocityProfile.vi"("Pose"=w559, "time"=w539, "intervalo"=w536, "estimatives"=w562, "Path  Smooth"=w560, "V_max"=w568, "Accel"=w567, "DesAccel"=w566) -> ("Time X"=w557:dbl[], "Velocities X"=w556:dbl[], "Time Y"=w555:dbl[], "Velocities Y"=w554:dbl[])  [unwired: 4 in]
                    n228 = call "VelocityCommand.vi"("intervalo"=w536, "estimatives"=w562, "Velocities Y"=w554, "Time Y"=w555, "Velocities X"=w556, "Time X"=w557) -> ("Vy"=w553:dbl, "Vx"=w552:dbl)  [unwired: 4 in]
                    n229 = feedback-in #27(w536) -> ()
                    n230 = call "VelocityControl.vi"("estimatives"=w562, "Dest_orientation"=w561, "Position"=w559, "Waypoint 1"=w549, "Waypoint 0"=w546, "Vx"=w552, "Vy"=w553, "output xy"=w563, "output inc"=w565, "output angle"=w564) -> ("Output Velocity"=w558:dbl[])  [unwired: 5 in]
                  }
                  frame True {
                  }
                }
                n231 = feedback-in #25(w522) -> ()
                n232 = Index Array(array=w521) -> (element #1=w526:dbl, element #2=w525:dbl, element #3=w524:dbl)  [unwired: 3 in]
              }
              frame 9 {
                n233 = Not A Number/Path/Refnum?(number/path/refnum=w572) -> (NaN/Path/Refnum?=w571:bool[][])
                n234 = Or Array Elements(Boolean array=w571) -> (logical OR=w570:bool)
                n235 = feedback #28() -> (w573:dbl[])  [unwired: 1 in]
                n236 = case shown="False" w570 {
                  tunnel: w587 -> [w620 _]
                  tunnel: w586 -> [w619 _]
                  tunnel: w585 -> [w618 _]
                  tunnel: w584 -> [w617 _]
                  tunnel: w583 -> [w616 _]
                  tunnel: w582 -> [w615 _]
                  tunnel: w581 -> [w614 _]
                  tunnel: w580 -> [w613 _]
                  tunnel: w572 -> [w612 _]
                  tunnel: w579 -> [w611 _]
                  tunnel: [w610 w621] -> w574
                  tunnel: w575 -> [w597 _]
                  tunnel: w573 -> [_ w621]
                  frame False {
                    # "dt = t2 -t1"
                    n237 = call "GetTimeInSeconds.vi"("Timestamp"=w597) -> ("Numeric"=w591:dbl)  [unwired: 10 in]
                    n238 = feedback-in #29(w591) -> ()
                    n239 = feedback #29(0.0 ("Numeric")) -> (w590:dbl)
                    n240 = Index Array(array=w612) -> (element #1=w599:dbl[], element #2=w602:dbl[])  [unwired: 4 in]
                    n241 = Subtract(x=w591, y=w590) -> (x-y=w593:dbl)
                    n242 = Empty Array?(array=w599) -> (empty?=w600:bool)
                    n243 = feedback #30(0.015 ("Numeric")) -> (w592:dbl)
                    n244 = Select(t=w611, s=w600, f=w599) -> (s? t:f=w598:dbl[])
                    n245 = Empty Array?(array=w602) -> (empty?=w603:bool)
                    n246 = Equal?(x=w593, y=0.0) -> (x = y?=w596:bool)
                    n247 = Select(t=w598, s=w603, f=w602) -> (s? t:f=w601:dbl[])
                    n248 = Select(t=w592, s=w596, f=w593) -> (s? t:f=w588:dbl)
                    n249 = call "PathVelocityProfile.vi"("Pose"=w611, "time"=w591, "intervalo"=w588, "estimatives"=w614, "Path  Smooth"=w612, "V_max"=w620, "Accel"=w619, "DesAccel"=w618) -> ("Time X"=w609:dbl[], "Velocities X"=w608:dbl[], "Time Y"=w607:dbl[], "Velocities Y"=w606:dbl[])  [unwired: 4 in]
                    n250 = call "VelocityCommand.vi"("intervalo"=w588, "estimatives"=w614, "Velocities Y"=w606, "Time Y"=w607, "Velocities X"=w608, "Time X"=w609) -> ("Vy"=w605:dbl, "Vx"=w604:dbl)  [unwired: 4 in]
                    n251 = feedback-in #30(w588) -> ()
                    n252 = call "VelocityControl.vi"("estimatives"=w614, "Dest_orientation"=w613, "Position"=w611, "Waypoint 1"=w601, "Waypoint 0"=w598, "Vx"=w604, "Vy"=w605, "output xy"=w615, "output inc"=w617, "output angle"=w616) -> ("Output Velocity"=w610:dbl[])  [unwired: 5 in]
                  }
                  frame True {
                  }
                }
                n253 = feedback-in #28(w574) -> ()
                n254 = Index Array(array=w573) -> (element #1=w578:dbl, element #2=w577:dbl, element #3=w576:dbl)  [unwired: 3 in]
              }
              frame 10 {
                n255 = Not A Number/Path/Refnum?(number/path/refnum=w624) -> (NaN/Path/Refnum?=w623:bool[][])
                n256 = Or Array Elements(Boolean array=w623) -> (logical OR=w622:bool)
                n257 = feedback #31() -> (w625:dbl[])  [unwired: 1 in]
                n258 = case shown="False" w622 {
                  tunnel: w639 -> [w672 _]
                  tunnel: w638 -> [w671 _]
                  tunnel: w637 -> [w670 _]
                  tunnel: w636 -> [w669 _]
                  tunnel: w635 -> [w668 _]
                  tunnel: w634 -> [w667 _]
                  tunnel: w633 -> [w666 _]
                  tunnel: w632 -> [w665 _]
                  tunnel: w624 -> [w664 _]
                  tunnel: w631 -> [w663 _]
                  tunnel: [w662 w673] -> w626
                  tunnel: w627 -> [w649 _]
                  tunnel: w625 -> [_ w673]
                  frame False {
                    # "dt = t2 -t1"
                    n259 = call "GetTimeInSeconds.vi"("Timestamp"=w649) -> ("Numeric"=w643:dbl)  [unwired: 10 in]
                    n260 = feedback-in #32(w643) -> ()
                    n261 = feedback #32(0.0 ("Numeric")) -> (w642:dbl)
                    n262 = Index Array(array=w664) -> (element #1=w651:dbl[], element #2=w654:dbl[])  [unwired: 4 in]
                    n263 = Subtract(x=w643, y=w642) -> (x-y=w645:dbl)
                    n264 = Empty Array?(array=w651) -> (empty?=w652:bool)
                    n265 = feedback #33(0.015 ("Numeric")) -> (w644:dbl)
                    n266 = Select(t=w663, s=w652, f=w651) -> (s? t:f=w650:dbl[])
                    n267 = Empty Array?(array=w654) -> (empty?=w655:bool)
                    n268 = Equal?(x=w645, y=0.0) -> (x = y?=w648:bool)
                    n269 = Select(t=w650, s=w655, f=w654) -> (s? t:f=w653:dbl[])
                    n270 = Select(t=w644, s=w648, f=w645) -> (s? t:f=w640:dbl)
                    n271 = call "PathVelocityProfile.vi"("Pose"=w663, "time"=w643, "intervalo"=w640, "estimatives"=w666, "Path  Smooth"=w664, "V_max"=w672, "Accel"=w671, "DesAccel"=w670) -> ("Time X"=w661:dbl[], "Velocities X"=w660:dbl[], "Time Y"=w659:dbl[], "Velocities Y"=w658:dbl[])  [unwired: 4 in]
                    n272 = call "VelocityCommand.vi"("intervalo"=w640, "estimatives"=w666, "Velocities Y"=w658, "Time Y"=w659, "Velocities X"=w660, "Time X"=w661) -> ("Vy"=w657:dbl, "Vx"=w656:dbl)  [unwired: 4 in]
                    n273 = feedback-in #33(w640) -> ()
                    n274 = call "VelocityControl.vi"("estimatives"=w666, "Dest_orientation"=w665, "Position"=w663, "Waypoint 1"=w653, "Waypoint 0"=w650, "Vx"=w656, "Vy"=w657, "output xy"=w667, "output inc"=w669, "output angle"=w668) -> ("Output Velocity"=w662:dbl[])  [unwired: 5 in]
                  }
                  frame True {
                  }
                }
                n275 = feedback-in #31(w626) -> ()
                n276 = Index Array(array=w625) -> (element #1=w630:dbl, element #2=w629:dbl, element #3=w628:dbl)  [unwired: 3 in]
              }
            }
          }
          frame True {
            w674 = 0.0 ("output")
          }
        }
        n277 = Bundle By Name(cluster=w86, "v_tangent"=w71, "v_normal"=w70, "v_ang"=w66) -> (w85:T2)
      }
      n278 = Bundle By Name(cluster=w33, "our_robots"=w34) -> (w32:T1)
    }
    frame True {
      n279 = call "potential-field.vi"("IA State Output in"=w676) -> ("IA State Output out"=w675:T1)  [unwired: 10 in]
    }
  }
  n280 = Unbundle By Name(w7) -> ("IA Judge.command enum"=w6:T10)
  n281 = Equal?(x=w6, y=Command_Enum."Halt") -> ()  [unwired: 1 out]
  n282 = Or(x="Debug", y=FALSE) -> (x .or. y?=w4:bool)
  n283 = case shown="True" w4 {
    tunnel: [w677 w682] -> w8
    tunnel: w7 -> [w677 w679]
    tunnel: "IA State Output in" -> [_ w680]
    frame False {
    }
    frame True {
      n284 = Unbundle By Name(w679) -> ("our_robots"=w678:T2[])
      n285 = for {
        tunnel: [w685] -> w681 mode=indexing
        tunnel: w678 -> [w683] mode=indexing
        w684 = 0.0 ("v_normal")
        n286 = Bundle By Name(cluster=w683, "v_tangent"=w684, "v_normal"=w684, "v_ang"=w684) -> (w685:T2)
      }
      n287 = Bundle By Name(cluster=w680, "our_robots"=w681) -> (w682:T1)
    }
  }
  "IA State Output out" <- w8
